vi "Calculate Partial S Parameters.vi"(0 "Standard Data":T1[](array[typedef]), 5 "Result Data":T1[](array[typedef]), 11 "error in (no error)":errorcluster) -> (4 "S Parameters":cdb[][](array[numeric]), 15 "error out":errorcluster)   [LabVIEW 2023, in "RFFixtureCharact.Public.lvlib" / "Vector Abstract Path.lvclass"]
uses:
  Vector Abstract Path.lvclass
  Instruments/Cal Standard/Type Definitions/One-Port Charact Data.ctl
  Instruments/Cal Standard/Type Definitions/Standard Type.ctl
  <vilib>/Analysis/7linalg.llb/Solve Complex Linear Equations (single right hand).vi
  Vector Abstract Path.lvclass/Vector Abstract Path.ctl
  <vilib>/Analysis/NI_AALPro.lvlib
  Instruments/Cal Standard/Cal Standard Base/Cal Standard Base.lvclass
  Instruments/RFFixtureCharact.Instruments.lvlib
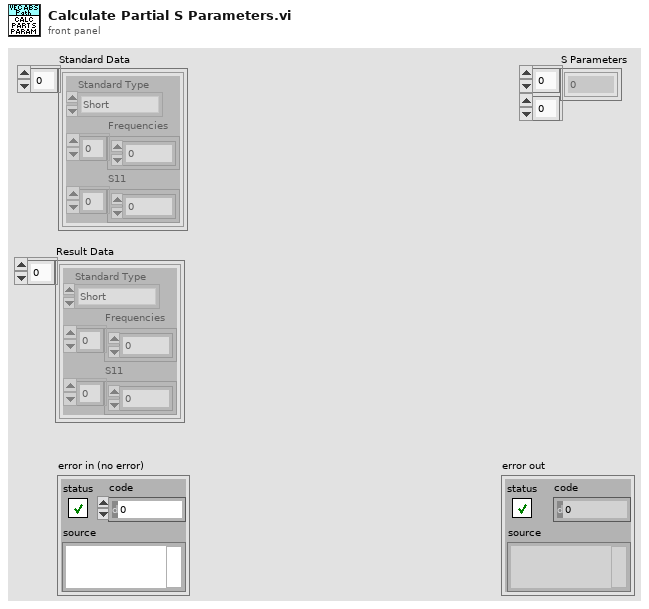
[diagram p1: front panel]
types:
  T1 = typedef "RFFixtureCharact.Instruments.lvlib/One-Port Charact Data.ctl" = cluster{"Standard Type":T2, "Frequencies":dbl[], "S11":cdb[]}
  T2 = typedef "RFFixtureCharact.Instruments.lvlib/Standard Type.ctl" = enum16{"Short", "Open", "Load", "PowerMeter", "None"}
  T3 = typedef "NI_Matrix.lvlib/ComplexMatrix.ctl" = cdb[][]
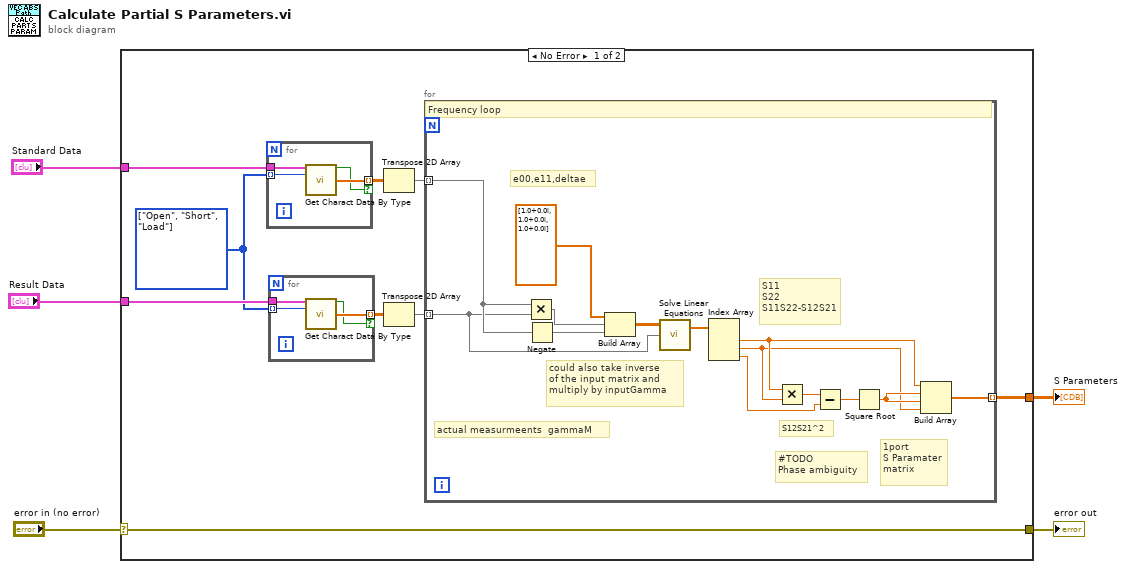
[diagram p0: block diagram]
diagram:
  n1 = case shown="No Error" "error in (no error)" {
    selector: "error in (no error)" -> [w14 w37]
    tunnel: [w14 w37] -> w4
    tunnel: "Standard Data" -> [w13 _]
    tunnel: "Result Data" -> [w12 _]
    tunnel: [w6 _] -> w1
    frame No Error {
      w11 = T2[] [enum."Open", enum."Short", enum."Load"] items=["Short", "Open", "Load", "PowerMeter", "None"]
      n2 = for {
        tunnel: w13 -> [w22]
        tunnel: w11 -> [w21] mode=indexing
        tunnel: [w20] -> w10 mode=indexing if=w19
        n3 = call "Get Charact Data By Type.vi"("Charact Data"=w22, "Standard Type"=w21) -> ("Found"=w19:bool, "S11"=w20:cdb[])  [unwired: 11 in, 1 out]
      }
      n4 = for {
        tunnel: w12 -> [w18]
        tunnel: w11 -> [w17] mode=indexing
        tunnel: [w16] -> w8 mode=indexing if=w15
        n5 = call "Get Charact Data By Type.vi"("Charact Data"=w18, "Standard Type"=w17) -> ("Found"=w15:bool, "S11"=w16:cdb[])  [unwired: 11 in, 1 out]
      }
      n6 = Transpose 2D Array(2D array=w10) -> (transposed array=w9:cdb[][])
      n7 = Transpose 2D Array(2D array=w8) -> (transposed array=w7:cdb[][])
      n8 = for {
        tunnel: [w27] -> w6 mode=indexing
        tunnel: w9 -> [w24] mode=indexing
        tunnel: w7 -> [w23] mode=indexing
        # "1port \nS Paramater\nmatrix"
        # "S12S21^2"
        # "could also take inverse\nof the input matrix and\nmultiply by inputGamma"
        # "actual measurmeents  gammaM"
        # "e00,e11,deltae"
        # "#TODO\nPhase ambiguity"
        # "S11\nS22\nS11S22-S12S21"
        # "Frequency loop"
        n9 = Multiply(x=w24, y=w23) -> (x*y=w34:cdb[])
        n10 = Negate(x=w24) -> (-x=w35:cdb[])
        n11 = Build Array(cdb[] [1.0+0.0i, 1.0+0.0i, 1.0+0.0i], w34, w35) -> (w26:T3)
        n12 = call-poly <vilib>:"Solve Linear Equations.vi"("Known Vector"=w23, "Input Matrix"=w26) -> ("Solution Vector"=w25:cdb[])  [unwired: 1 in, 1 out]
        n13 = Index Array(array=w25) -> (element #1=w29:cdb, element #2=w28:cdb, element #3=w32:cdb)  [unwired: 3 in]
        n14 = Multiply(x=w29, y=w28) -> (x*y=w33:cdb)
        n15 = Subtract(x=w33, y=w32) -> (x-y=w31:cdb)
        n16 = Square Root(x=w31) -> (sqrt(x)=w30:cdb)
        n17 = Build Array(w29, w30, w30, w28) -> (w27:cdb[])
      }
    }
    frame Error {
    }
  }
  "error out" <- w4
  "S Parameters" <- w1
